vi "Set Channel Names and Default Values from Slot.vi"(8 "error in":errorcluster, 9 "default values":dbl[](array[numeric]), 10 "channel names":string[](array[string]), 11 "slot ref in":T1 format="%.0x") -> (0 "error out":errorcluster, 3 "slot ref out":T1 format="%.0x")   [LabVIEW 2017, in "Scan Engine Scripting.lvlib"]
uses:
  <vilib>/NI Veristand/Custom Device API/Custom Device Item Ref.ctl
  Scan Engine Scripting.lvlib
  <vilib>/NI Veristand/Custom Device Tools/Custom Device Utility Library/Custom Device Utility Library.lvlib
  <vilib>/NI Veristand/Custom Device API/Custom Device API.lvlib
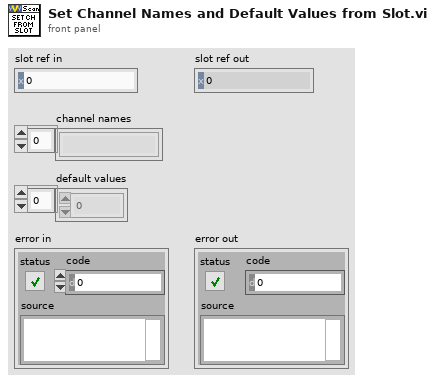
[diagram p1: front panel]
types:
  T1 = typedef "Custom Device API.lvlib/Custom Device Item Ref.ctl" = u64
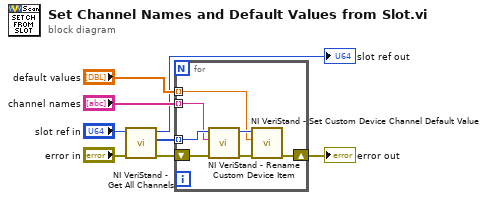
[diagram p0: block diagram]
diagram:
  n1 = call <vilib>:"NI VeriStand - Get All Channels.vi"("error in"="error in", "Section Ref in"="slot ref in") -> ("error out"=w4:errorcluster, "Channel Refs"=w3:T1[], "Section Ref out"=→"slot ref out":T1)  [unwired: 6 in, 1 out]
  n2 = for {
    tunnel: w3 -> [w14] mode=indexing
    tunnel: "channel names" -> [w13] mode=indexing
    shift-right: [w10] -> w7
    shift-left: w4 -> [w15]
    tunnel: "default values" -> [w9] mode=indexing
    n3 = call <vilib>:"NI VeriStand - Rename Custom Device Item.vi"("error in (no error)"=w15, "New Name"=w13, "Item Ref in"=w14) -> ("error out"=w11:errorcluster, "Item Ref out"=w12:T1)  [unwired: 6 in, 1 out]
    n4 = call <vilib>:"NI VeriStand - Set Custom Device Channel Default Value.vi"("error in (no error)"=w11, "Default Value"=w9, "Channel Ref in"=w12) -> ("error out"=w10:errorcluster)  [unwired: 7 in, 1 out]
  }
  "error out" <- w7
